vi "CSM - Forward States to CSM.vi"(6 "High Priority(T)":bool=TRUE, 7 "Module Name":string, 8 "Error In (no error)":errorcluster, 11 "State(s) in (\"\")":string) -> (0 "error out":errorcluster)   [LabVIEW 2020, in "Communicable State Machine.lvlib"]
doc: "Request CSM to Post a message to CSM specified. This is usually used in sub-loops with a CSM for acting as a holistic module.\n\n<b>Inputs:</b>\n - <b>Status</b>: Message to post.\n - <b>Arguments (\"\")</b>: Argument of the message.\n - <b>Target Module</b>:Target CSM module name.\n - <b>Module Name</b>:Host Module Name\n - <b>Error In (no error)</b>: Error cluster\n\n<b>Outputs:</b>\n - <b>error out</b>: Error cluster"
uses:
  Communicable State Machine.lvlib
  _CSM_MSG_TYPE.ctl
  _Cross CSM State Data.ctl
  _Cross CSM State Response.ctl
  _CSM_Response Source Message.ctl
  _CSMOFGVOPER.ctl
  Priority Queue.lvclass/Priority Queue.ctl
  Priority Queue.lvclass
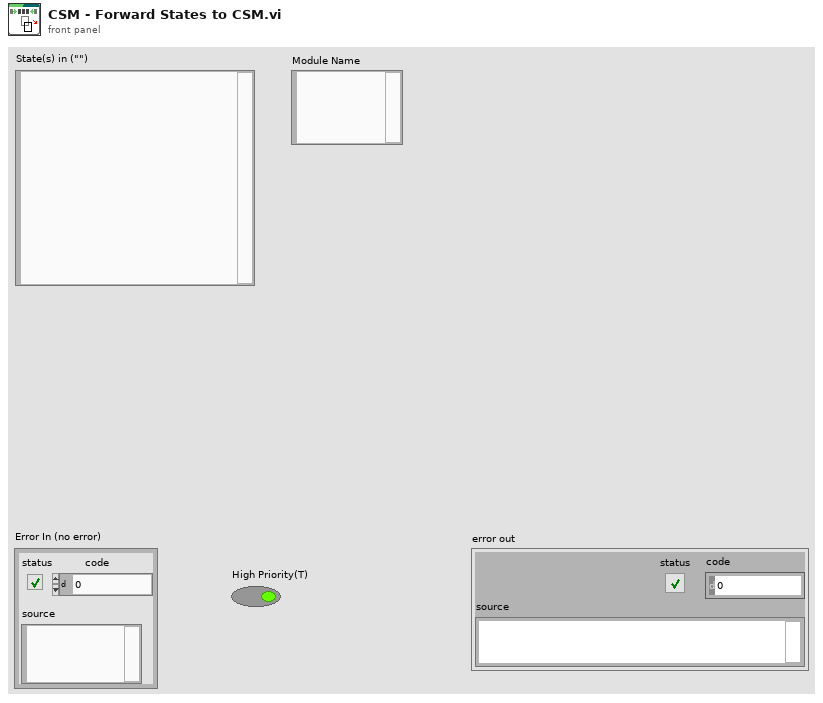
[diagram p1: front panel]
types:
  T1 = typedef "Communicable State Machine.lvlib/_CSM_MSG_TYPE.ctl" = enum16{"Sync Message(-@)", "Async Message(->)", "Async without Response(->|)", "Async Response", "Broadcast(-><all>)", "Broadcast(-><status>)", "Broadcast(-><interrupt>)", "Append to JKISM States", "Append to JKISM States(High Priority)"}
  T2 = typedef "Communicable State Machine.lvlib/_Cross CSM State Data.ctl" = cluster{"Msg Type":T1, "state":string, "args":string, "source":string, "RespQ":refnum<queue>, "Response For Message":T3, "Target":string}
  T3 = typedef "Communicable State Machine.lvlib/_CSM_Response Source Message.ctl" = cluster{"‘State":string, "’Arguments":string, "’Error":errorcluster}
  T4 = typedef "Communicable State Machine.lvlib/_CSMOFGVOPER.ctl" = enum16{"Create If not Exist", "Get By Name", "List", "Check If Name Exists", "Release", "Module Status", "Create Status Event Handler", "Destroy Status Event Handler"}
  T5 = typedef "Communicable State Machine.lvlib/_CSMObj.ctl" = cluster{"Requested Name":string, "Module Name":string, "Mode":T6, "Queue":refnum<class "Priority Queue.lvclass">, "CSM-Data":refnum<data-value>, "User Event":refnum<user-event>, "Status Change Event":refnum<user-event>, "Allowed Messages":string[], "Mode-Data":refnum<data-value>, "Group Name":string, "Exit Event":refnum<user-event>}
  T6 = typedef "Communicable State Machine.lvlib/_CSM_MODE.ctl" = enum16{"Not Exist", "Stand Alone", "CSM", "Worker Agent", "Worker", "Chain", "Chain Node"}
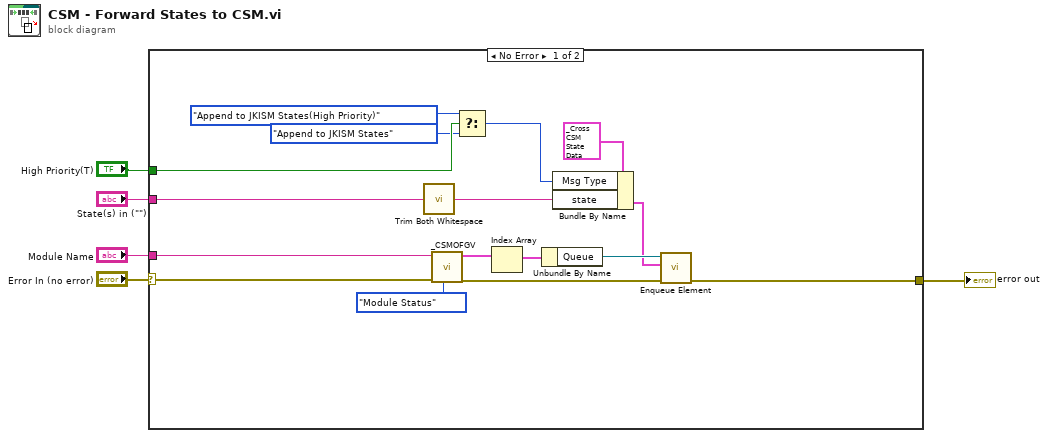
[diagram p0: block diagram]
diagram:
  n1 = case shown="No Error" "Error In (no error)" {
    selector: "Error In (no error)" -> [w20 w22]
    tunnel: "State(s) in (\"\")" -> [w19 _]
    tunnel: [w21 w22] -> w3
    tunnel: "Module Name" -> [w18 _]
    tunnel: "High Priority(T)" -> [w17 _]
    frame No Error {
      n2 = call "Trim Both Whitespace.vi"("string"=w19) -> ("trimmed string"=w16:string)  [unwired: 1 in]
      n3 = call "_CSMOFGV.vi"("Operation"=_CSMOFGVOPER."Module Status", "Error in"=w20, "Name(\"\" to use uuid) in"=w18) -> ("Error out"=w9:errorcluster, "Array"=w14:T5[])  [unwired: 6 in, 1 out]
      n4 = Select(t=_CSM_MSG_TYPE."Append to JKISM States(High Priority)" ("Msg Type"), s=w17, f=_CSM_MSG_TYPE."Append to JKISM States" ("Msg Type")) -> (s? t:f=w8:T1)
      n5 = Index Array(array=w14) -> (element=w13:T5)  [unwired: 1 in]
      n6 = Unbundle By Name(w13) -> ("Queue"=w12:refnum<class "Priority Queue.lvclass">)
      n7 = Bundle By Name(cluster=T2 {"Msg Type"=enum."Sync Message(-@)", "state"="", "args"="", "source"="", "RespQ"=refnum, "Response For Message"={"‘State"="", "’Arguments"="", "’Error"={"status"=FALSE, "code"=0, "source"=""}}, "Target"=""} ("element"), "Msg Type"=w8, "state"=w16) -> (w10:T2)
      n8 = call "Enqueue Element.vi"("error in (no error)"=w9, "Cross JKI State Machine State"=w10, "Priority Queue"=w12) -> ("error out"=w21:errorcluster)  [unwired: 7 in, 1 out]
    }
    frame Error {
    }
  }
  "error out" <- w3
